vi "Gesha_UTS2.vi"() -> ()   [LabVIEW 2020]
panel:
  out "Number of Errors":i32
  out "WARNING":bool
  in  "HIGH Limit":dbl(slide) scale=0.0..100.0
  in  "LOW Limit":dbl(slide) scale=0.0..100.0
  in  "Operator":string
  out "Waveform Chart":T1(graph)
  out "START/STOP":bool
  in  "STOP":bool
  in  "START/STOP":bool
  in  "C   or   F":bool
  in  "Filename":path
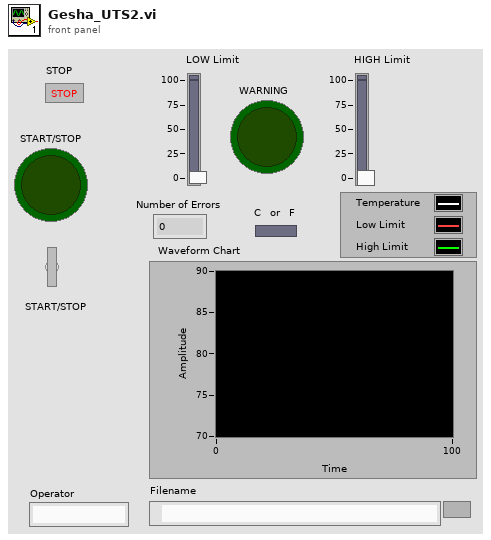
[diagram p1: front panel]
types:
  T1 = cluster{"Temperature (deg F)":dbl, "LOW Limit":dbl, "HIGH Limit":dbl}
  T2 = enum16{"open", "replace", "create", "open or create", "replace or create", "replace or create with confirmation"}
  T3 = cluster{"Y":dbl, "LOW Limit":dbl, "HIGH Limit":dbl}
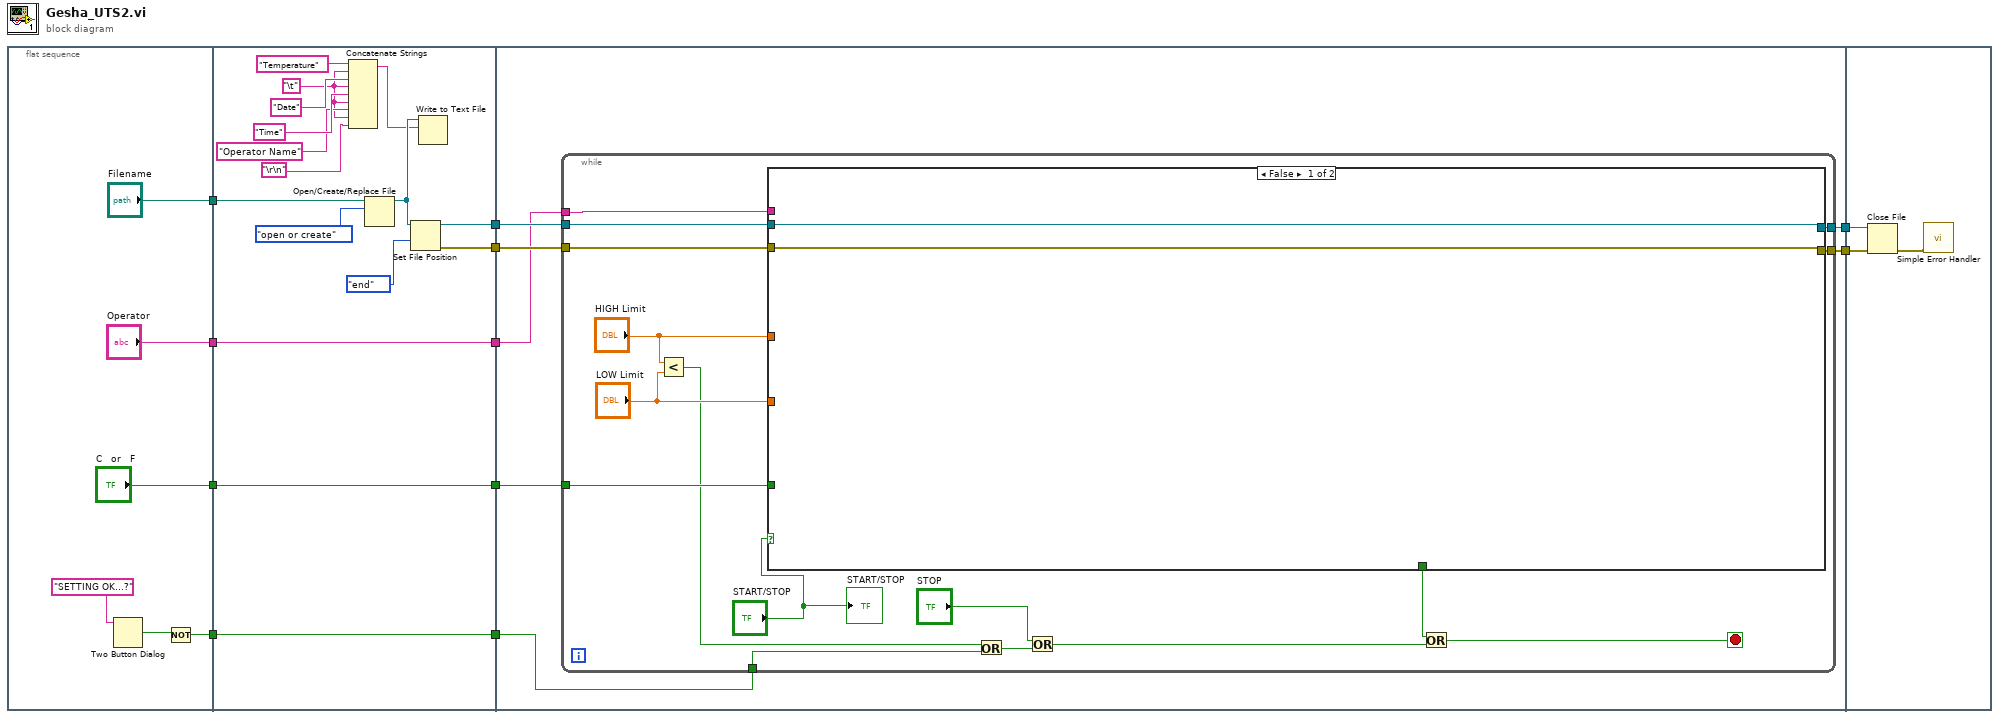
[diagram p0: block diagram]
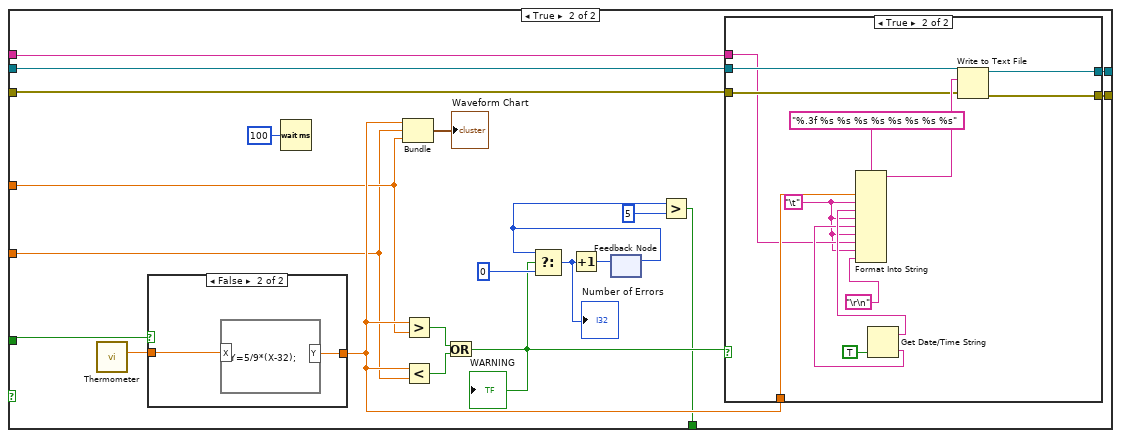
[diagram p2: hidden frame]
diagram:
  n1 = flat-sequence {
    tunnel: ["Filename"] -> w11
    tunnel: ["C   or   F"] -> w9
    tunnel: [w13] -> w7
    tunnel: ["Operator"] -> w1
    tunnel: w11 -> [w33]
    tunnel: [w31] -> w10
    tunnel: w9 -> [w31]
    tunnel: [w30] -> w8
    tunnel: w7 -> [w30]
    tunnel: [w29] -> w6
    tunnel: [w28] -> w5
    tunnel: [w25] -> w2
    tunnel: w1 -> [w25]
    tunnel: w10 -> [w40]
    tunnel: w8 -> [w39]
    tunnel: w6 -> [w38]
    tunnel: w5 -> [w37]
    tunnel: [w36] -> w4
    tunnel: [w35] -> w3
    tunnel: w2 -> [w34]
    tunnel: w4 -> [w100]
    tunnel: w3 -> [w99]
    frame #0 {
      n2 = Two Button Dialog(message="SETTING OK...?") -> (T button?=w14:bool)  [unwired: 2 in]
      n3 = Not(x=w14) -> (.not. x?=w13:bool)
    }
    frame #1 {
      w18 = "\t"
      n4 = Concatenate Strings("Temperature" ("string"), w18, "Date" ("string"), w18, "Time" ("string"), w18, "Operator Name" ("string"), w18, "\r\n") -> (w24:string)
      n5 = Open/Create/Replace File(file path (use dialog)=w33, operation (0:open)=T2."open or create") -> (refnum out=w27:refnum<file>)  [unwired: 4 in, 2 out]
      n6 = Set File Position(refnum=w27, from (0:start)=enum16{"start", "end", "current"}."end") -> (refnum out=w29:refnum<file>, error out=w28:errorcluster)  [unwired: 2 in]
      n7 = Write to Text File(file (use dialog)=w27, text=w24) -> ()  [unwired: 2 in, 3 out]
    }
    frame #2 {
      n8 = while {
        tunnel: w40 -> [w56]
        tunnel: w39 -> [w55]
        tunnel: w38 -> [w54]
        tunnel: w37 -> [w53]
        tunnel: [w52] -> w36
        tunnel: [w51] -> w35
        tunnel: w34 -> [w50]
        stop <- w45 stop-if-true
        n9 = Less?(x="HIGH Limit", y="LOW Limit") -> (x < y?=w41:bool)
        n10 = case shown="False" "START/STOP" {
          tunnel: w56 -> [_ w79]
          tunnel: w54 -> [w58 w74]
          tunnel: w53 -> [w57 w73]
          tunnel: [w58 w72] -> w52
          tunnel: [w57 w71] -> w51
          tunnel: w50 -> [_ w70]
          tunnel: "HIGH Limit" -> [_ w67]
          tunnel: "LOW Limit" -> [_ w66]
          tunnel: [_ w60] -> w44
          frame False {
          }
          frame True {
            n11 = call "Thermometer.vi"() -> ("Temperature (deg F)"=w68:dbl)  [unwired: 1 in]
            n12 = case shown="False" w79 {
              tunnel: w68 -> [w95 w97]
              tunnel: [w95 w96] -> w69
              frame True {
              }
              frame False {
                n13 = formula code="Y=5/9*(X-32);"("X"=w97) -> ("Y"=w96:dbl)
              }
            }
            n14 = Wait (ms)(milliseconds to wait=u32 100) -> ()  [unwired: 1 out]
            n15 = Bundle("Y"=w69, "LOW Limit"=w66, "HIGH Limit"=w67) -> (→"Waveform Chart":T3)  [unwired: 1 in]
            n16 = Greater?(x=w69, y=w67) -> (0:w78:bool)
            n17 = Less?(x=w69, y=w66) -> (x < y?=w77:bool)
            n18 = Or(x=w78, y=w77) -> (x .or. y?=w61:bool)
            "WARNING" <- w61
            n19 = feedback #1() -> (w65:i32)  [unwired: 1 in]
            n20 = Select(t=w65, s=w61, f=0) -> (s? t:f=w59:i32)
            "Number of Errors" <- w59
            n21 = Increment(x=w59) -> (x+1=w62:i32)
            n22 = feedback-in #1(w62) -> ()
            n23 = Greater?(x=w65, y=5) -> (0:w60:bool)
            n24 = case shown="True" w61 {
              tunnel: w69 -> [_ w93]
              tunnel: w74 -> [w80 w91]
              tunnel: w73 -> [w81 w90]
              tunnel: [w80 w89] -> w72
              tunnel: [w81 w88] -> w71
              tunnel: w70 -> [_ w83]
              frame False {
              }
              frame True {
                w82 = "\t"
                n25 = Get Date/Time String(want seconds? (F)=TRUE) -> (date string=w86:string, time string=w85:string)  [unwired: 2 in]
                n26 = Format Into String "Format Into String"(format string="%.3f %s %s %s %s %s %s %s %s", w93, w82, w86, w82, w85, w82, w83, w82, "\r\n") -> (resulting string=w92:string)  [unwired: 2 in, 1 out]
                n27 = Write to Text File(file (use dialog)=w91, text=w92, error in=w90) -> (refnum out=w89:refnum<file>, error out=w88:errorcluster)  [unwired: 1 in, 1 out]
              }
            }
          }
        }
        n28 = Or(x=w41, y=w55) -> (x .or. y?=w49:bool)
        n29 = Or(x="STOP", y=w49) -> (x .or. y?=w46:bool)
        n30 = Or(x=w44, y=w46) -> (x .or. y?=w45:bool)
        "START/STOP" <- "START/STOP"
      }
    }
    frame #3 {
      n31 = Close File(refnum=w100, error in=w99) -> (error out=w98:errorcluster)  [unwired: 1 out]
      n32 = call <vilib>:"Simple Error Handler.vi"("error in (no error)"=w98) -> ()  [unwired: 4 in, 5 out]
    }
  }
